vi "testare_retea.vi"() -> ()   [LabVIEW 2024]
uses:
  <vilib>/National Instruments/NI Super Simple Neural Networks/Neural Network.lvclass
panel:
  out "Valoare":dbl
  out "Ghicire":string
  out "Image":T1(plugin-control)
  in  "path to PNG file":path
  in  "stop":bool
  out "litera ghicita":cluster{string, "Numeric Control":dbl}[](array[cluster]) {"Numeric Control" scale=0.0..1.0}
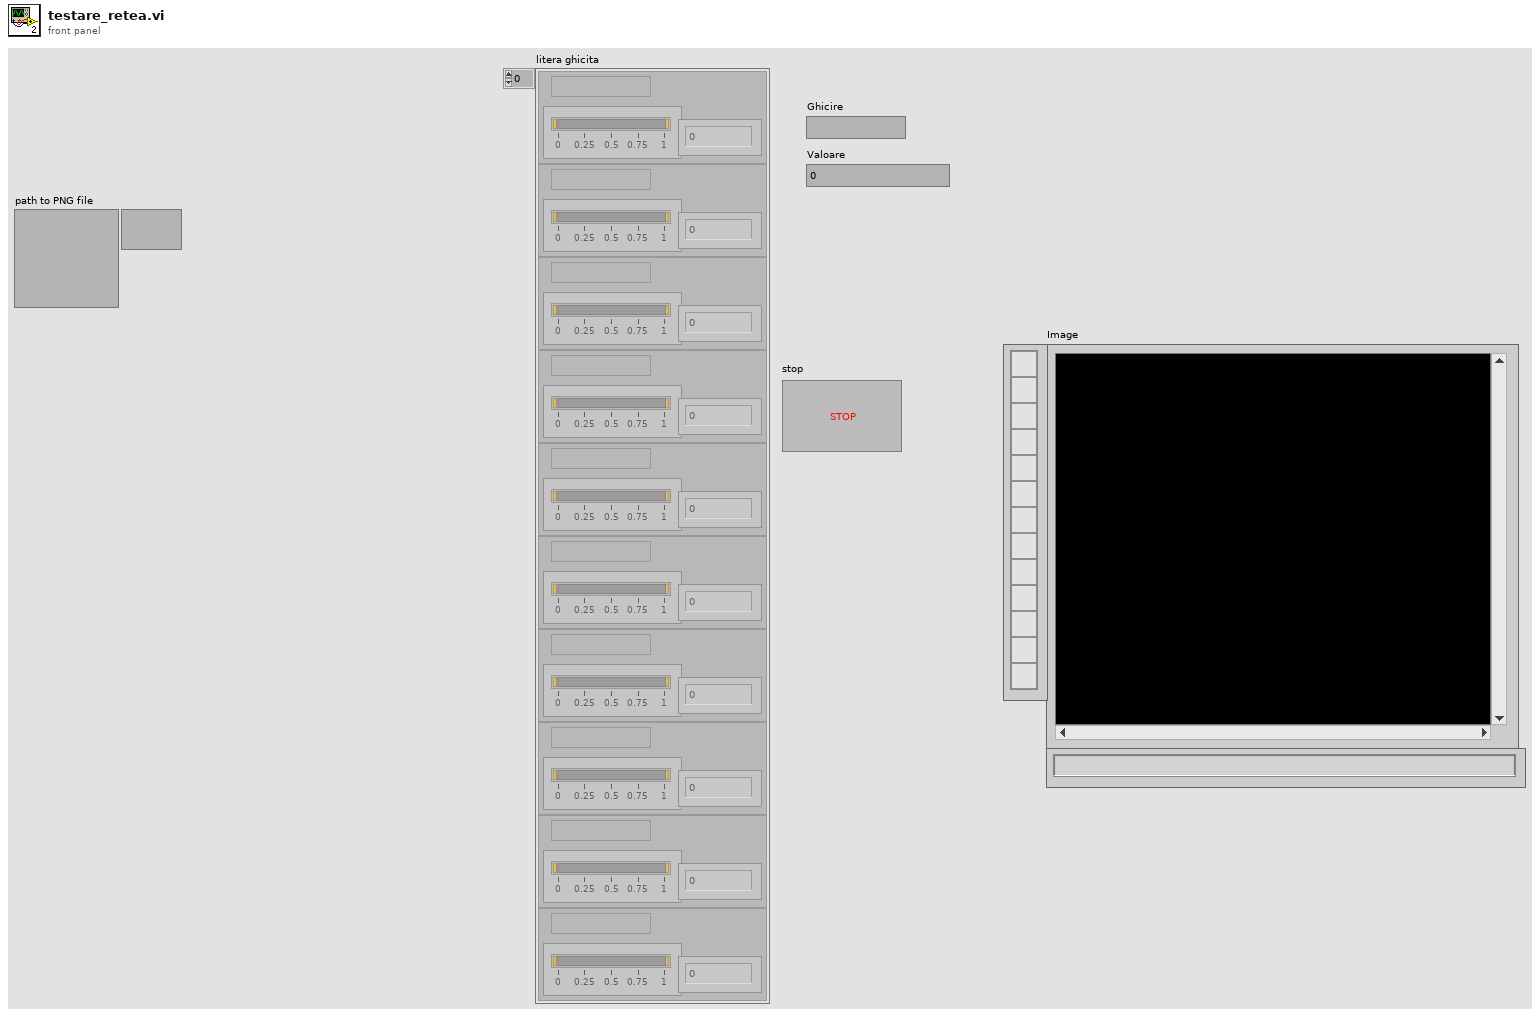
[diagram p1: front panel]
types:
  T1 = typedef "IMAQ Image.ctl" = refnum<image>
  T2 = typedef "imagedata.ctl" = cluster{"image type":i32, "image depth":i32, "image":u8[], "mask":u8[], "colors":u32[], "Rectangle":cluster{"left":i16, "top":i16, "right":i16, "bottom":i16}}
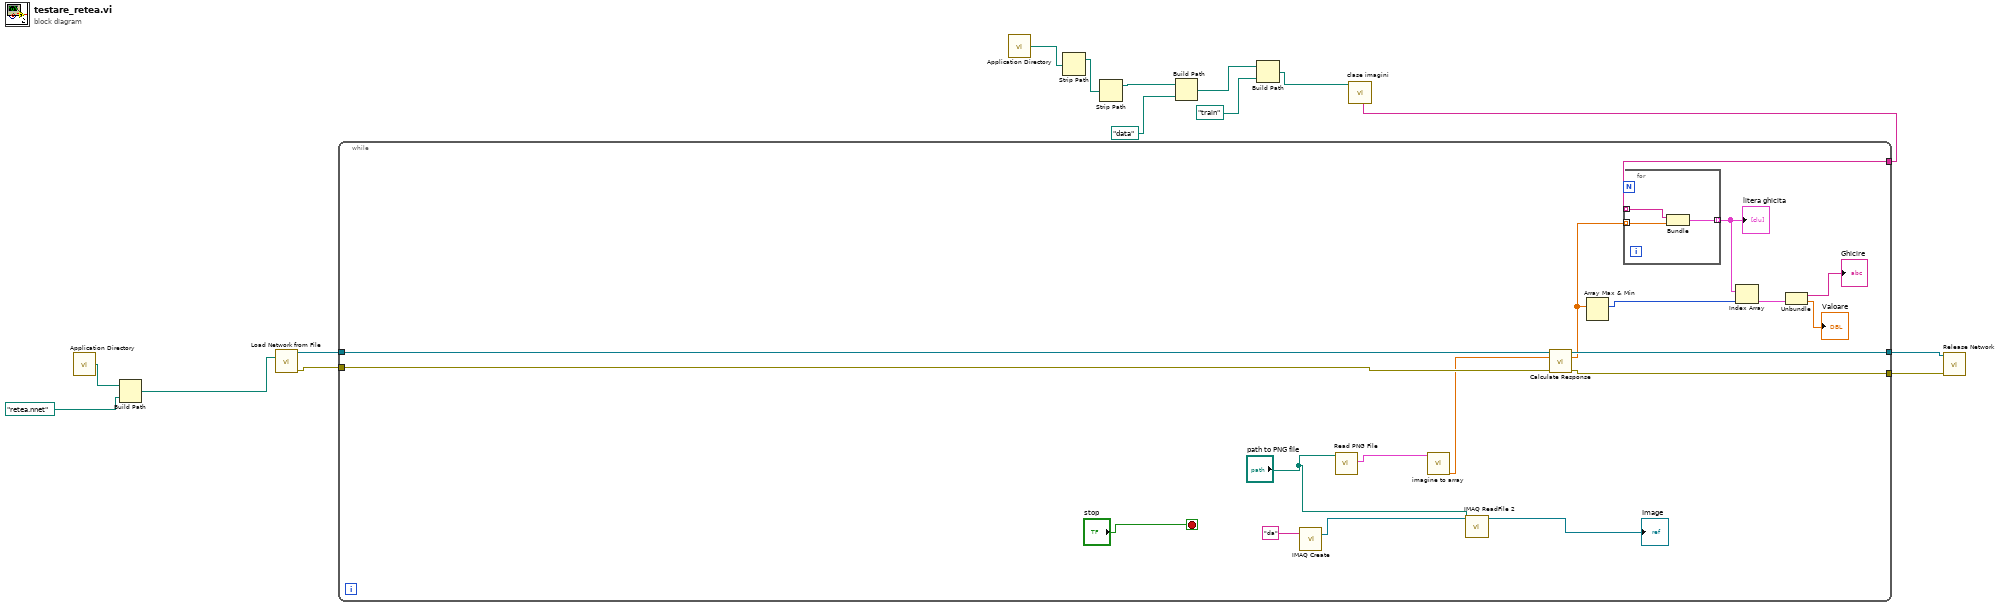
[diagram p0: block diagram]
diagram:
  n1 = call <vilib>:"Application Directory.vi"() -> ("Application Directory"=w11:path)
  n2 = Build Path(base path=w11, name or relative path=path "retea.nnet") -> (appended path=w10:path)
  n3 = call <vilib>:"Load Network from File.vi"("File Path (dialog)"=w10) -> ("Neural Network Out"=w15:refnum<class "Neural Network.lvclass">, "Error Out"=w14:errorcluster)  [unwired: 11 in, 2 out]
  n4 = call <vilib>:"Application Directory.vi"() -> ("Application Directory"=w5:path)
  n5 = Strip Path(path=w5) -> (stripped path=w6:path)  [unwired: 1 out]
  n6 = Strip Path(path=w6) -> (stripped path=w7:path)  [unwired: 1 out]
  n7 = Build Path(base path=w7, name or relative path=path "data") -> (appended path=w8:path)
  n8 = Build Path(base path=w8, name or relative path=path "train") -> (appended path=w1:path)
  n9 = call "clase imagini.vi"("dataset folder"=w1) -> ("nume clase"=w2:string[])  [unwired: 10 in]
  n10 = while {
    tunnel: w15 -> [w33]
    tunnel: w14 -> [w32]
    tunnel: [w31] -> w13
    tunnel: [w30] -> w12
    tunnel: w2 -> [w22]
    stop <- "stop" stop-if-true
    n11 = call "IMAQ Create"("Image Name"="da") -> ("New Image"=w27:T1)  [unwired: 4 in, 1 out]
    n12 = call <vilib>:"Read PNG File.vi"("path to PNG file"="path to PNG file") -> ("image data"=w28:T2)  [unwired: 8 in, 2 out]
    n13 = call "imagine to array.vi"("image data"=w28) -> ("array imagine"=w29:dbl[])  [unwired: 9 in, 1 out]
    n14 = call "IMAQ ReadFile 2"("File Path"="path to PNG file", "Image"=w27) -> ("Image Out"=→"Image":T1)  [unwired: 5 in, 4 out]
    n15 = call <vilib>:"Calculate Response.vi"("Neural Network In"=w33, "Inputs"=w29, "Error In"=w32) -> ("Neural Network Out"=w31:refnum<class "Neural Network.lvclass">, "Outputs"=w23:dbl[], "Error Out"=w30:errorcluster)  [unwired: 10 in]
    n16 = Array Max & Min(array=w23) -> (max index (indices)=w18:i32)  [unwired: 3 out]
    n17 = for {
      tunnel: w23 -> [w36] mode=indexing
      tunnel: w22 -> [w35] mode=indexing
      tunnel: [w34] -> w21 mode=indexing
      n18 = Bundle(w35, "Numeric Control"=w36) -> (w34:cluster{string, "Numeric Control":dbl})  [unwired: 1 in]
    }
    "litera ghicita" <- w21
    n19 = Index Array "Index Array"(array=w21, index=w18) -> (element=w20:cluster{string, "Numeric Control":dbl})
    n20 = Unbundle(w20) -> (→"Ghicire":string, "Numeric Control"=→"Valoare":dbl)
  }
  n21 = call <vilib>:"Release Network.vi"("Neural Network"=w13, "Error In"=w12) -> ()  [unwired: 13 in, 1 out]
